vi "TCL Close.vi"(3 "Event File Refnum":refnum<k1>) -> ()   [LabVIEW 2009]
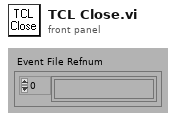
[diagram p1: front panel]
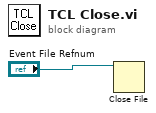
[diagram p0: block diagram]
diagram:
  n1 = Close File(refnum="Event File Refnum") -> ()  [unwired: 1 in, 2 out]
